vi "Read Chip ID.vi"(7 "SlaveID":u8, 8 "error in (no error)":errorcluster, 11 ".NET Refnum in":refnum<k24>) -> (0 "error out":errorcluster, 2 "32bit integer":i32[](array[numeric]), 3 ".NET Refnum out":refnum<k24>)   [LabVIEW 2017]
uses:
  C:/Users/chrisjan/Desktop/NowWorking/ITRI/DLL/Modbus.dll
  DLL/Modbus.dll
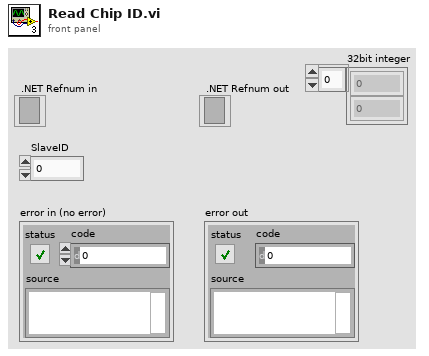
[diagram p1: front panel]
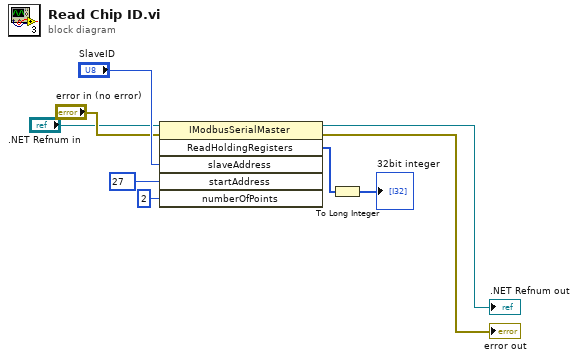
[diagram p0: block diagram]
diagram:
  n1 = invoke class="IModbusSerialMaster" method="ReadHoldingRegisters"(reference=".NET Refnum in", error in="error in (no error)", "slaveAddress"="SlaveID", "startAddress"=u16 27, "numberOfPoints"=u16 2) -> (reference out=→".NET Refnum out":refnum<k24>, error out=→"error out":errorcluster, "ReadHoldingRegisters"=w2:u16[])  [unwired: 1 in, 3 out]
  n2 = To Long Integer(number=w2) -> (32bit integer=→"32bit integer":i32[])
